vi "unique tagging query builder.vi"() -> ()   [LabVIEW 2021]
panel:
  in  "gathered spreadsheet string":string="14\tsw\tsw\taddons\t\tlvrtmod\t\t\t\n16\tacad\tsw\tappsw\t\tmultisim\t\t\t\n2695\tacad\t\t\t\t\t\t\t\n2710\tsw\tsw\tade\t\tlvbasefullpro\t\t\t\n2714\tsw2\t\t\t\t\t\t\t\n2719\tsw\tsw\tade\t\tlvbasefullpro\t\t\t\n2726\tembed\thw\t\t\tcriomod\t\tcurrent\t\n2733\tsw\tsw\taddons\t\tlvrtmod\t\t\t\n2734\tsw\tsw\tade\t\tlvbasefullpro\t\t\t\n2739\ttest\thw\tdevice\t\tinstctrl\t\t\t\n2744\tdaq\tsw\tade,syssw\tdriver\tdaqmx\t\t\t\n2751\tdaq\tsw\tsyssw\tdriver\tdaqmx\t\t\t\n2761\ttest\tsw\tsyssw\tdriver,3rdparty\tinstctrl\t\t\t\n2768\ttest\tsw\tsyssw\tdriver\thsdio\tcompat\t\t\n2776\ttest\thw\tmodule\t\tswitch\t\t\t\n2777\ttest\thw\tmodule\t\tswitch\t\t\t\n2781\ttest\thw\tmodule\t\tswitch\t\t\t\n2783\ttest\thw\tmodule\t\tswitch\t\t\t\n2785\ttest\thw\tmodule\t\tswitch\t\t\t\n2787\ttest\thw\tmodule\t\tswitch\t\t\t\n2799\ttest\thw\tmodule\t\tswitch\t\t\t\n2801\ttest\tsw\tsyssw\tdriver\tgpib\t\t\t\n2804\ttest\tsw\tsyssw\tdriver,3rdparty\tinstctrl\t\t\t\n2805\ttest\thw\tdevice\t\thsdio\t\t\t\n2816\ttest\tsw\tsyssw\tdriver,3rdparty\tinstctrl\t\t\tlinuxos\n"
  in  "Content Type":T1(ring)=enum."use DOCUMENTID"
  out "consolidated spreadsheet string":string
  # "Paste from spreadsheet.\nPaste should include DocID + all tag columns from portfolio, not including column headers.\nOutput will be minimum queries necessary versus tag combinations.\nYou can also just paste the GUIDs if you just need a good kSearch query\n***You will need to paste values into intermediate sheet and remove \"0\"s from cells if you're using my product tag lookup in your main spreadsheet."
  # "Copy to spreadsheet.\nAt most you will get columns for number of items in query, the concatenated tags used for comparison, the tag names for kSearch, and the queries themselves\nIf there are no tags above then you won't get any below\n***If it doesn't paste as expected, check your \"Text to Columns\" settings and make sure they're simply default Tab delimited. If you have been doing custom Text to Columns operations, it might affect the way it handles the incoming clipboard during the paste."
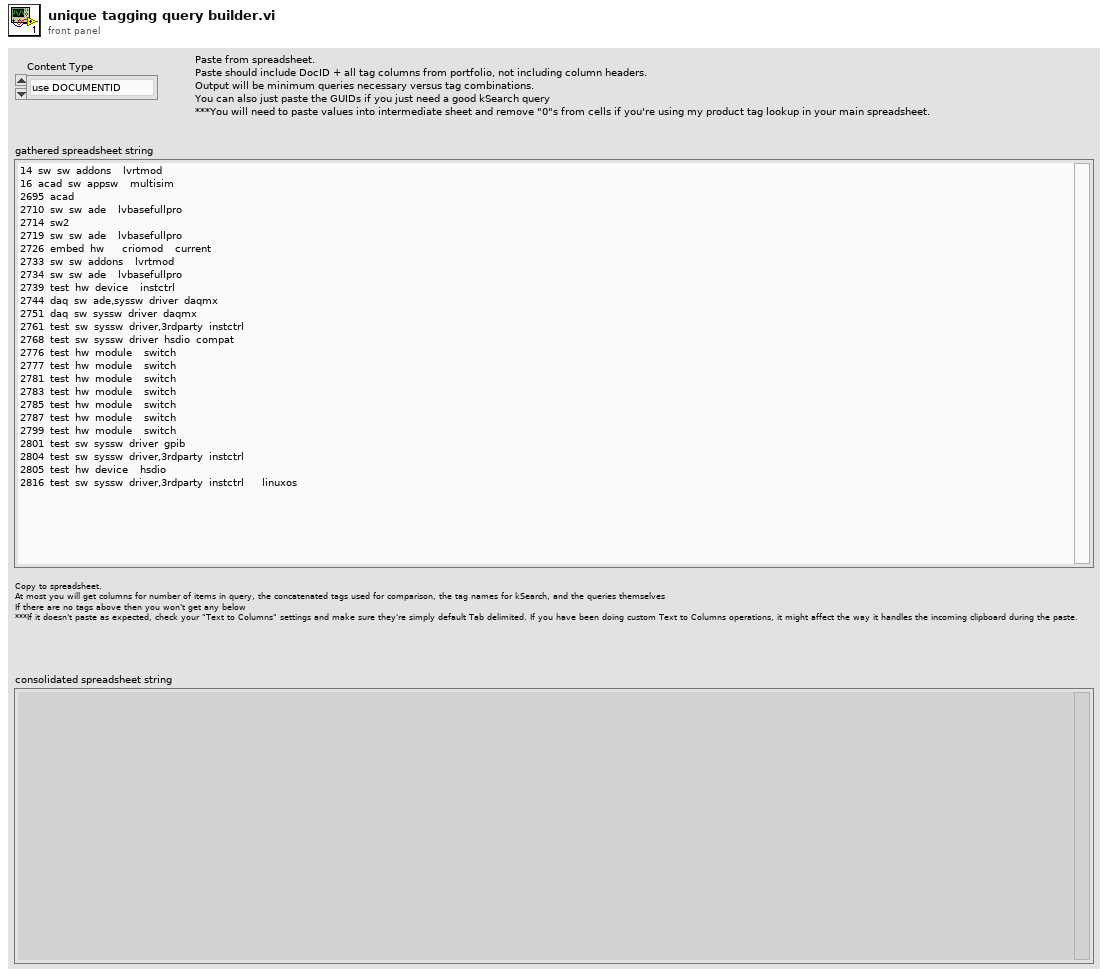
[diagram p1: front panel]
types:
  T1 = enum16{"Notes KB", "VCM Example", "Community Example", "Product Doc", "PSP", "Tutorial", "WP", "SFDC KB", "use URI", "use DOCUMENTID"}
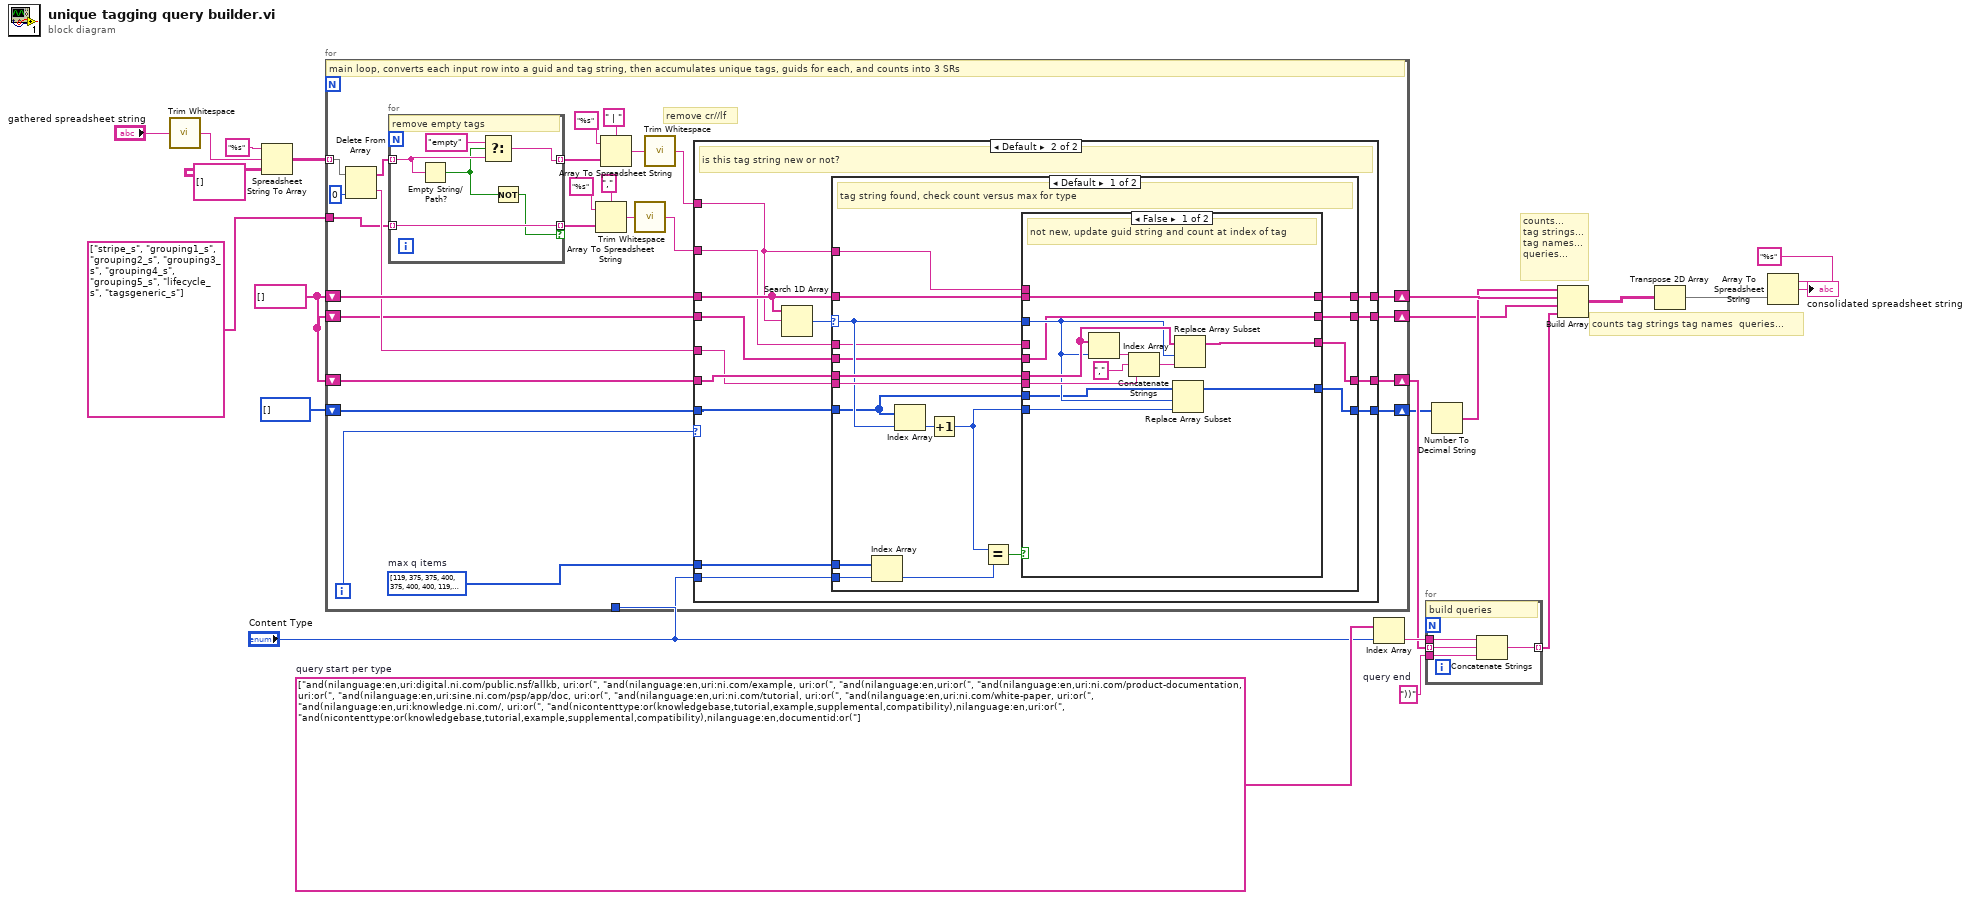
[diagram p0: block diagram]
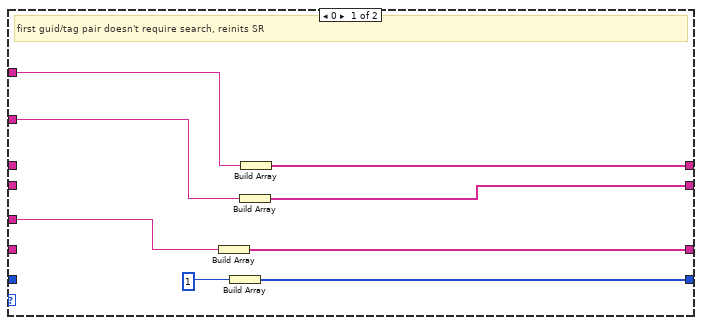
[diagram p2: hidden frame]
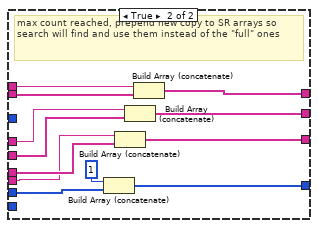
[diagram p3: hidden frame]
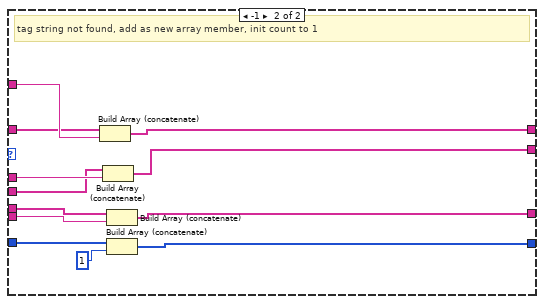
[diagram p4: hidden frame]
diagram:
  w17 = "))"  # query end
  w21 = string[] ["and(nilanguage:en,uri:digital.ni.com/public.nsf/allkb, uri:or(", "and(nilanguage:en,uri:ni.com/example, uri:or(", "and(nilanguage:en,uri:or(", "and(nilanguage:en,uri:ni.com/product-documentation, uri:or(", "and(nilanguage:en,uri:sine.ni.com/psp/app/doc, uri:or(", "and(nilanguage:en,uri:ni.com/tutorial, uri:or(", "and(nilanguage:en,uri:ni.com/white-paper, uri:or(", "and(nilanguage:en,uri:knowledge.ni.com/, uri:or(", "and(nicontenttype:or(knowledgebase,tutorial,example,supplemental,compatibility),nilanguage:en,uri:or(", "and(nicontenttype:or(knowledgebase,tutorial,example,supplemental,compatibility),nilanguage:en,documentid:or("]  # query start per type
  w3 = string[] []
  # "counts tag strings tag names  queries..."
  # "counts...\ntag strings...\ntag names...\nqueries..."
  n1 = call <vilib>:"Trim Whitespace.vi"("string"="gathered spreadsheet string") -> ("trimmed string"=w5:string)  [unwired: 1 in]
  n2 = Spreadsheet String To Array(format string="%s", spreadsheet string=w5, array type (2D Dbl)=string[][] []) -> (array=w7:string[][])  [unwired: 1 in]
  n3 = for {
    tunnel: w7 -> [w46] mode=indexing
    shift-right: [w43] -> w20
    shift-left: w3 -> [w42]
    shift-right: [w41] -> w18
    shift-left: w3 -> [w39]
    shift-right: [w35] -> w12
    shift-left: i32[] [] -> [w34]
    tunnel: "Content Type" -> [w32]
    tunnel: string[] ["stripe_s", "grouping1_s", "grouping2_s", "grouping3_s", "grouping4_s", "grouping5_s", "lifecycle_s", "tagsgeneric_s"] -> [w31]
    shift-right: [w23] -> w1
    shift-left: w3 -> [w24]
    i -> [w44]
    w33 = i32[] [119, 375, 375, 400, 375, 400, 400, 119, 119, 119]  # max q items
    # "remove cr//lf"
    # "main loop, converts each input row into a guid and tag string, then accumulates unique tags, guids for each, and counts into 3 SRs"
    n4 = Delete From Array(array=w46, index=0 ("disabled index (col)")) -> (deleted portion=w40:string, array with subset deleted=w38:string[])  [unwired: 1 in]
    n5 = for {
      tunnel: w38 -> [w130] mode=indexing
      tunnel: [w128] -> w48 mode=indexing
      tunnel: w31 -> [w127] mode=indexing
      tunnel: [w127] -> w26 mode=indexing if=w125
      # "remove empty tags"
      n6 = Empty String/Path?(string/path=w130) -> (empty?=w126:bool)
      n7 = Select(t="empty", s=w126, f=w130) -> (s? t:f=w128:string)
      n8 = Not(x=w126) -> (.not. x?=w125:bool)
    }
    n9 = Array To Spreadsheet String(delimiter (Tab)=",", array=w26, 3:"%s" ("format string")) -> (spreadsheet string=w28:string)
    n10 = Array To Spreadsheet String(delimiter (Tab)=" | ", array=w48, 3:"%s" ("format string")) -> (spreadsheet string=w37:string)
    n11 = call <vilib>:"Trim Whitespace.vi"("string"=w28) -> ("trimmed string"=w25:string)  [unwired: 1 in]
    n12 = call <vilib>:"Trim Whitespace.vi"("string"=w37) -> ("trimmed string"=w36:string)  [unwired: 1 in]
    n13 = case shown="Default" w44 {
      tunnel: [w55 w67] -> w43
      tunnel: w36 -> [w56 w68]
      tunnel: w42 -> [_ w69]
      tunnel: [w53 w64] -> w41
      tunnel: w40 -> [w54 w65]
      tunnel: w39 -> [_ w66]
      tunnel: [w51 w62] -> w35
      tunnel: w34 -> [_ w63]
      tunnel: w33 -> [_ w61]
      tunnel: w32 -> [_ w60]
      tunnel: w25 -> [w50 w58]
      tunnel: w24 -> [_ w59]
      tunnel: [w49 w57] -> w23
      frame 0 {
        # "first guid/tag pair doesn't require search, reinits SR"
        n14 = Build Array(w54) -> (w53:string[])
        n15 = Build Array(1) -> (w51:i32[])
        n16 = Build Array(w50) -> (w49:string[])
        n17 = Build Array(w56) -> (w55:string[])
      }
      frame Default {
        # "is this tag string new or not?"
        n18 = Search 1D Array(1D array=w69, element=w68) -> (index of element=w70:i32)  [unwired: 1 in]
        n19 = case shown="Default" w70 {
          selector: w70 -> [w77 _]
          tunnel: w69 -> [w84 w123]
          tunnel: w68 -> [w80 w124]
          tunnel: [w83 w122] -> w67
          tunnel: w66 -> [w79 w121]
          tunnel: w65 -> [w78 w120]
          tunnel: [w82 w119] -> w64
          tunnel: w63 -> [w76 w118]
          tunnel: [w81 w117] -> w62
          tunnel: w61 -> [w87 _]
          tunnel: w60 -> [w86 _]
          tunnel: w59 -> [w72 w114]
          tunnel: w58 -> [w73 w115]
          tunnel: [w71 w113] -> w57
          frame Default {
            # "tag string found, check count versus max for type"
            n20 = Index Array(array=w87, index=w86) -> (element=w74:i32)
            n21 = Index Array(array=w76, index=w77) -> (element=w88:i32)
            n22 = Increment(x=w88) -> (x+1=w75:i32)
            n23 = Equal?(x=w75, y=w74) -> (x = y?=w85:bool)
            n24 = case shown="False" w85 {
              tunnel: [w100 w110] -> w83
              tunnel: w84 -> [w100 w111]
              tunnel: [w93 w107] -> w82
              tunnel: [w92 w104] -> w81
              tunnel: w80 -> [_ w112]
              tunnel: w79 -> [w96 w109]
              tunnel: w78 -> [w95 w108]
              tunnel: w77 -> [w94 _]
              tunnel: w76 -> [w91 w106]
              tunnel: w75 -> [w90 _]
              tunnel: w73 -> [_ w103]
              tunnel: w72 -> [w89 w102]
              tunnel: [w89 w101] -> w71
              frame False {
                # "not new, update guid string and count at index of tag"
                n25 = Index Array(array=w96, index=w94) -> (element=w99:string)
                n26 = Concatenate Strings(w99, "," ("string"), w95) -> (w97:string)
                n27 = Replace Array Subset(array=w91, new element=w90, index=w94) -> (w92:i32[])
                n28 = Replace Array Subset(array=w96, new element=w97, index=w94) -> (w93:string[])
              }
              frame True {
                # "max count reached, prepend new copy to SR arrays so search will find and use them instead of the \"full\" ones"
                n29 = Build Array (concatenate)(1, w106) -> (w104:i32[])
                n30 = Build Array (concatenate)(w108, w109) -> (w107:string[])
                n31 = Build Array (concatenate)(w103, w102) -> (w101:string[])
                n32 = Build Array (concatenate)(w112, w111) -> (w110:string[])
              }
            }
          }
          frame -1 {
            # "tag string not found, add as new array member, init count to 1"
            n33 = Build Array (concatenate)(w123, w124) -> (w122:string[])
            n34 = Build Array (concatenate)(w114, w115) -> (w113:string[])
            n35 = Build Array (concatenate)(w121, w120) -> (w119:string[])
            n36 = Build Array (concatenate)(w118, 1) -> (w117:i32[])
          }
        }
      }
    }
  }
  n37 = Index Array(array=w21, index="Content Type") -> (element=w19:string)
  n38 = for {
    tunnel: w19 -> [w134]
    tunnel: w17 -> [w133]
    tunnel: w18 -> [w132] mode=indexing
    tunnel: [w131] -> w2 mode=indexing
    # "build queries"
    n39 = Concatenate Strings(w134, w132, w133) -> (w131:string)
  }
  n40 = Number To Decimal String(number=w12) -> (decimal integer string=w11:string[])  [unwired: 1 in]
  n41 = Build Array(w11, w20, w1, w2) -> (w22:string[][])
  n42 = Transpose 2D Array(2D array=w22) -> (transposed array=w16:string[][])
  n43 = Array To Spreadsheet String(array=w16, 3:"%s" ("format string")) -> (spreadsheet string=→"consolidated spreadsheet string":string)  [unwired: 1 in]
